vi "Vision Data.vi"() -> ()   [LabVIEW 2013]
panel:
  out "Number of Particles":dbl
  out "Distance (in)":dbl
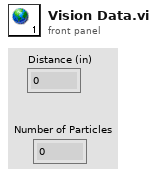
[diagram p1: front panel]
diagram:
